vi "ASDA-A2_Disconnect.vi"(8 "error in":errorcluster, 11 "Buffer Data In":T1) -> (0 "error out":errorcluster, 3 "Buffer Data Out":T1)   [LabVIEW 2016]
uses:
  Data Def/ASDA-A2_Buffer Data.ctl
  <vilib>/Modbus/master/Modbus Master.lvclass
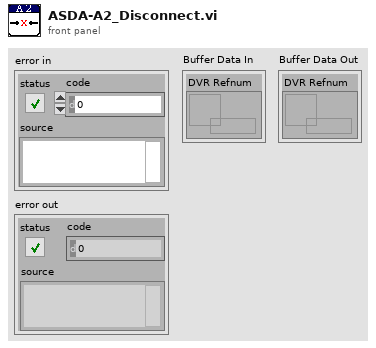
[diagram p1: front panel]
types:
  T1 = typedef "ASDA-A2_Buffer Data.ctl" = cluster{"DVR Refnum":refnum<data-value>}
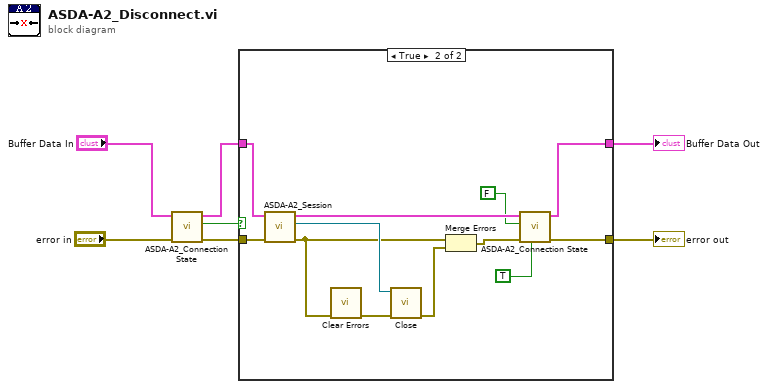
[diagram p0: block diagram]
diagram:
  n1 = call "ASDA-A2_Connection State.vi"("error in"="error in", "Buffer Data In"="Buffer Data In") -> ("error out"=w3:errorcluster, "State Out"=w1:bool, "Buffer Data Out"=w2:T1)  [unwired: 7 in]
  n2 = case shown="True" w1 {
    tunnel: [w9 w11] -> w7
    tunnel: [w8 w15] -> w6
    tunnel: w3 -> [w8 w17]
    tunnel: w2 -> [w9 w16]
    frame False {
    }
    frame True {
      n3 = call "ASDA-A2_Session.vi"("error in"=w17, "Buffer Data In"=w16) -> ("error out"=w19:errorcluster, "Session Out"=w20:refnum<class "Modbus Master.lvclass">, "Buffer Data Out"=w12:T1)  [unwired: 7 in]
      n4 = call <vilib>:"Clear Errors.vi"("error in (no error)"=w19) -> ("error out"=w21:errorcluster)  [unwired: 5 in, 1 out]
      n5 = call-dynamic "Close.vi"("error in (no error)"=w21, "Modbus master in"=w20) -> ("error out"=w18:errorcluster)  [unwired: 9 in]
      n6 = Merge Errors(w19, w18) -> (w14:errorcluster)
      n7 = call "ASDA-A2_Connection State.vi"("Get/Set (T=Set)"=TRUE, "error in"=w14, "State In"=FALSE, "Buffer Data In"=w12) -> ("error out"=w15:errorcluster, "Buffer Data Out"=w11:T1)  [unwired: 5 in, 1 out]
    }
  }
  "error out" <- w6
  "Buffer Data Out" <- w7
